vi "Configure Message.vi"(0 "VISA resource name":refnum<visa-resource-name>, 5 "Message Number (1)":i32=1 min=1 max=100 step=1, 7 "Message (\"\")":string, 11 "error in (no error)":errorcluster) -> (4 "VISA resource name out":refnum<visa-resource-name>, 6 "Message Number":i32, 15 "error out":errorcluster)   [LabVIEW 2020, in "Yokogawa GX Series.lvlib"]
doc: "Sets the message.\n\nCommand: SMessage"
uses:
  <instrlib>/Yokogawa GX Series/Yokogawa GX Series.lvlib
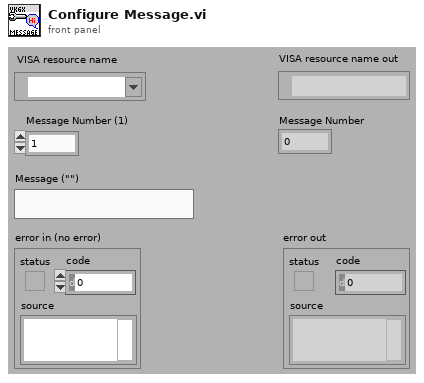
[diagram p1: front panel]
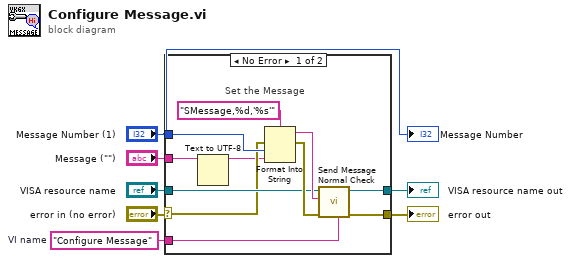
[diagram p0: block diagram]
diagram:
  w7 = "Configure Message"  # VI name
  n1 = case shown="No Error" "error in (no error)" {
    selector: "error in (no error)" -> [w10 w19]
    tunnel: w7 -> [w16 _]
    tunnel: "Message (\"\")" -> [w9 _]
    tunnel: "VISA resource name" -> [w14 w20]
    tunnel: [w13 w20] -> w4
    tunnel: [w12 w19] -> w3
    tunnel: "Message Number (1)" -> [w11 _]
    frame No Error {
      # "Set the Message"
      n2 = Text to UTF-8(11:w9) -> (3:w8:string)  [unwired: 2 in, 1 out]
      n3 = Format Into String(format string="SMessage,%d,'%s'", error in=w10, w11, w8) -> (resulting string=w15:string, error out=w17:errorcluster)  [unwired: 1 in]
      n4 = call <instrlib>:"Send Message Normal Check.vi"("Source (\"\")"=w16, "error in (no error)"=w17, "Send Message (\"\")"=w15, "VISA resource name"=w14) -> ("error out"=w12:errorcluster, "VISA resource name out"=w13:refnum<visa-resource-name>)  [unwired: 2 in, 4 out]
    }
    frame Error {
    }
  }
  "error out" <- w3
  "VISA resource name out" <- w4
  "Message Number" <- "Message Number (1)"
